vi "DEMO.vi"() -> ()   [LabVIEW 2013]
uses:
  Control/SW.ctl
  Control/Data.ctl
  Control/YV.ctl
  Control/State.ctl
panel:
  out "Data Out":T1
  in  "Start":bool
  in  "SW In":T3
  in  "停止":bool
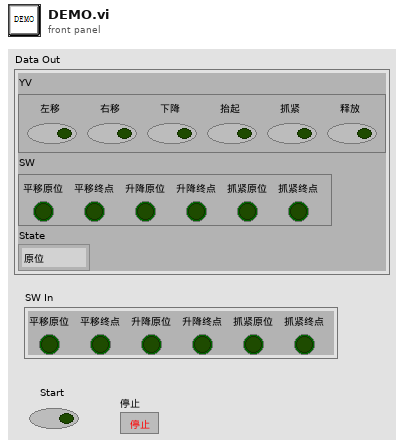
[diagram p1: front panel]
types:
  T1 = typedef "Data.ctl" = cluster{"YV":T2, "SW":T3, "State":T4}
  T2 = typedef "YV.ctl" = cluster{"左移":bool, "右移":bool, "下降":bool, "抬起":bool, "抓紧":bool, "释放":bool}
  T3 = typedef "SW.ctl" = cluster{"平移原位":bool, "平移终点":bool, "升降原位":bool, "升降终点":bool, "抓紧原位":bool, "抓紧终点":bool}
  T4 = typedef "State.ctl" = enum16{"原位", "A侧下降", "夹紧工件", "A侧抬起", "右移", "B侧下降", "释放工件", "B侧抬起", "左移"}
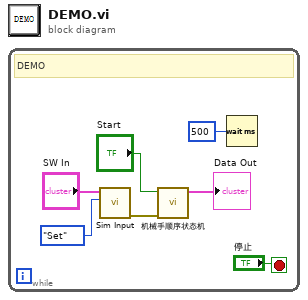
[diagram p0: block diagram]
diagram:
  n1 = while {
    stop <- "停止" stop-if-true
    # "DEMO"
    n2 = call "Sim Input.vi"("mode"=enum16{"Get", "Set"}."Set", "SW In"="SW In") -> ("error out"=w1:errorcluster)  [unwired: 7 in, 1 out]
    n3 = call "机械手顺序状态机.vi"("error in (no error)"=w1, "Start"="Start") -> ("Data Out"=→"Data Out":T1)  [unwired: 8 in, 1 out]
    n4 = Wait (ms)(milliseconds to wait=u32 500 ("等待时间（毫秒）")) -> ()  [unwired: 1 out]
  }
